vi "Asylum_Driver_LithographyInitialize.vi"(8 "error in (no error)":errorcluster, 11 "Background Image":path=path "Q:/inst/AFM Drift/SAA00010002.ibw") -> (0 "error out":errorcluster, 3 "Offset out":cluster{"X":dbl, "Y":dbl})   [LabVIEW 2019]
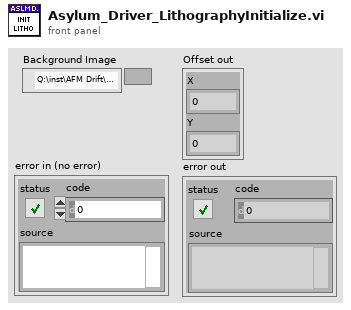
[diagram p1: front panel]
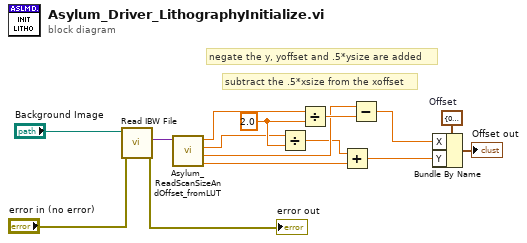
[diagram p0: block diagram]
diagram:
  w13 = 2.0
  w14 = cluster{"X":dbl, "Y":dbl} {"X"=0.0, "Y"=0.0}  # Offset
  # "subtract the .5*xsize from the xoffset"
  # "negate the y, yoffset and .5*ysize are added"
  n1 = call "Read IBW File.vi"("error in (no error)"="error in (no error)", "Path"="Background Image") -> ("error out"=→"error out":errorcluster, "Notes LUT"=w6:variant)  [unwired: 7 in, 1 out]
  n2 = call "Asylum_ReadScanSizeAndOffset_fromLUT.vi"("Notes LUT"=w6) -> ("Y Offset"=w4:dbl, "X Offset"=w5:dbl, "Y Range"=w2:dbl, "X Range"=w3:dbl)  [unwired: 7 in]
  n3 = Divide(x=w2, y=w13) -> (x/y=w1:dbl)
  n4 = Divide(x=w3, y=w13) -> (x/y=w12:dbl)
  n5 = Add(x=w1, y=w4) -> (x+y=w10:dbl)
  n6 = Subtract(x=w5, y=w12) -> (x-y=w11:dbl)
  n7 = Bundle By Name(cluster=w14, "X"=w11, "Y"=w10) -> (→"Offset out":cluster{"X":dbl, "Y":dbl})
